vi "oa_Reset if Parameters Change for Triggered Even Angle Signal (1 Channel).vi"(7 "reset? (T)":bool=TRUE, 8 "block size":i32=1024, 9 "trigger period [rev]":dbl=1.0, 11 "even angle signal":cluster{"r0":dbl, "dr":dbl, "Y":dbl[]}={"r0"=0.0, "dr"=1.0, "Y"=[]} {"r0" format="%.2p"; "dr" format="%.2p"; "Y" format="%.2f"}) -> (0 "block size out":i32, 1 "trigger period out [rev]":dbl, 3 "even angle signal out":cluster{"r0":dbl, "dr":dbl, "Y":dbl[]}={"r0"=0.0, "dr"=1.0, "Y"=[]} {"r0" format="%.2p"; "dr" format="%.2p"; "Y" format="%.2f"}, 5 "reset out":bool)   [LabVIEW 2017, in "SoundVib_OAUtility.lvlib"]
uses:
  <vilib>/addons/Sound and Vibration/Order Analysis/Utility/SoundVib_OAUtility.lvlib
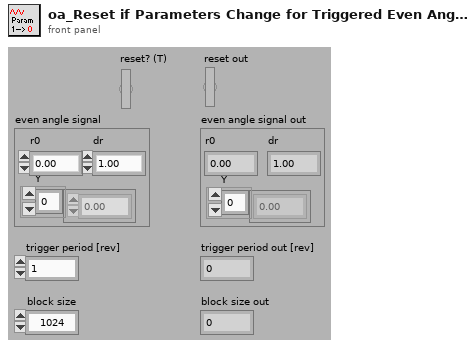
[diagram p1: front panel]
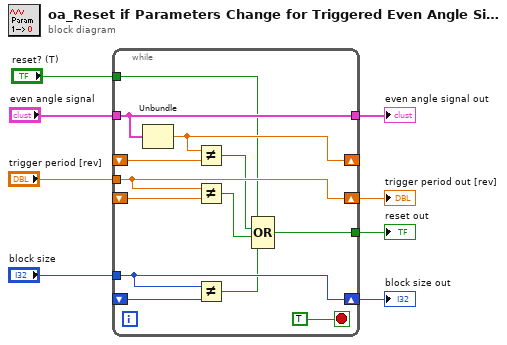
[diagram p0: block diagram]
diagram:
  n1 = while {
    tunnel: "even angle signal" -> [w14]
    tunnel: [w14] -> w1
    tunnel: "trigger period [rev]" -> [w20]
    tunnel: "block size" -> [w18]
    shift-right: [w20] -> w5
    shift-left: _ -> [w19]
    shift-right: [w18] -> w4
    shift-left: _ -> [w17]
    shift-right: [w13] -> _
    shift-left: _ -> [w12]
    tunnel: "reset? (T)" -> [w11]
    tunnel: [w9] -> w2
    stop <- TRUE stop-if-true
    n2 = Unbundle(w14) -> ("dr"=w13:dbl)  [unwired: 2 out]
    n3 = Not Equal?(x=w13, y=w12) -> (x != y?=w10:bool)
    n4 = Not Equal?(x=w20, y=w19) -> (x != y?=w15:bool)
    n5 = Not Equal?(x=w18, y=w17) -> (x != y?=w16:bool)
    n6 = Compound Arithmetic op=OR(w11, w10, w15, w16) -> (w9:bool)
  }
  "trigger period out [rev]" <- w5
  "block size out" <- w4
  "reset out" <- w2
  "even angle signal out" <- w1
